vi "MPB_signal_write_read.vi"(8 "error in":errorcluster, 10 "Send Commands":T4, 11 "RBS session in":T1) -> (0 "error out":errorcluster, 2 "MPB Status":T3 {"InletDCportNegLowRes (VDCportNeg)" format="%.2f"; "HeatgActv (HVIL FB)" format="%.2f"; "InletACportEgy (ACfuseNeg)" format="%.2f"; "InletDCportPosLowRes (VDCportPos)" format="%.2f"; "InletACportFuseLowRes (ACfusePos)" format="%.2f"; "DCbusVoltgUpprHalf" format="%.2f"; "Vac" format="%.2f"; "TrfmrTemp2" format="%.2f"; "TrfmrTemp1" format="%.2f"; "HAPSFltCode" format="%.2f"; "ACCurr4" format="%.2f"; "ACCurr3" format="%.2f"; "ACCurr2" format="%.2f"; "ACCurr1" format="%.2f"; "HAPSCurr" format="%.2f"; "HAPSFltFlag" format="%.2f"; "HAPSVoltgOut" format="%.2f"; "HwFltCode" format="%.2f"; "HwFltFlag" format="%.2f"; "HAPSVoltgIn" format="%.2f"; "BattPortPosFuseLowRes" format="%.2f"; "BattPortNegFuseLowRes" format="%.2f"; "BattPortVoltgLowRes" format="%.2f"; "DCbusVoltg" format="%.2f"; "DCbusVoltgLowrHalf" format="%.2f"; "InletDCportVoltgHiRes" format="%.2f"; "BattPortPower" format="%.2f"; "BattVoltgHiRes" format="%.2f"; "BattCurrDAB2" format="%.2f"; "BattCurrDAB1" format="%.2f"}, 3 "RBS session out":T1)   [LabVIEW 2020]
uses:
  controls/Send Commands.ctl
  controls/MPB Status.ctl
  <vilib>/AKKA/PROVEtech-RBS/private/RBS Session.ctl
  <vilib>/AKKA/PROVEtech-RBS/private/RBS Core/RBS Core Data.ctl
  <vilib>/AKKA/PROVEtech-RBS/private/RBS status.ctl
  <vilib>/AKKA/PROVEtech-RBS/SubVIs/Write (Signals Single-point).vi
  <vilib>/AKKA/PROVEtech-RBS/SubVIs/Read (Signals Single-point).vi
  <vilib>/AKKA/PROVEtech-RBS/PROVEtechRBS.lvlib
panel:
  # "Other"
  # "AC Port Info"
  # "Battery Port Info"
  # "Fault Info"
  # "1"
  # "2"
  # "3"
  # "4"
  # "5"
  # "6"
  # "7"
  # "DC Bus Info"
  # "HAPS Info"
  # "Temps"
  # "1"
  # "2"
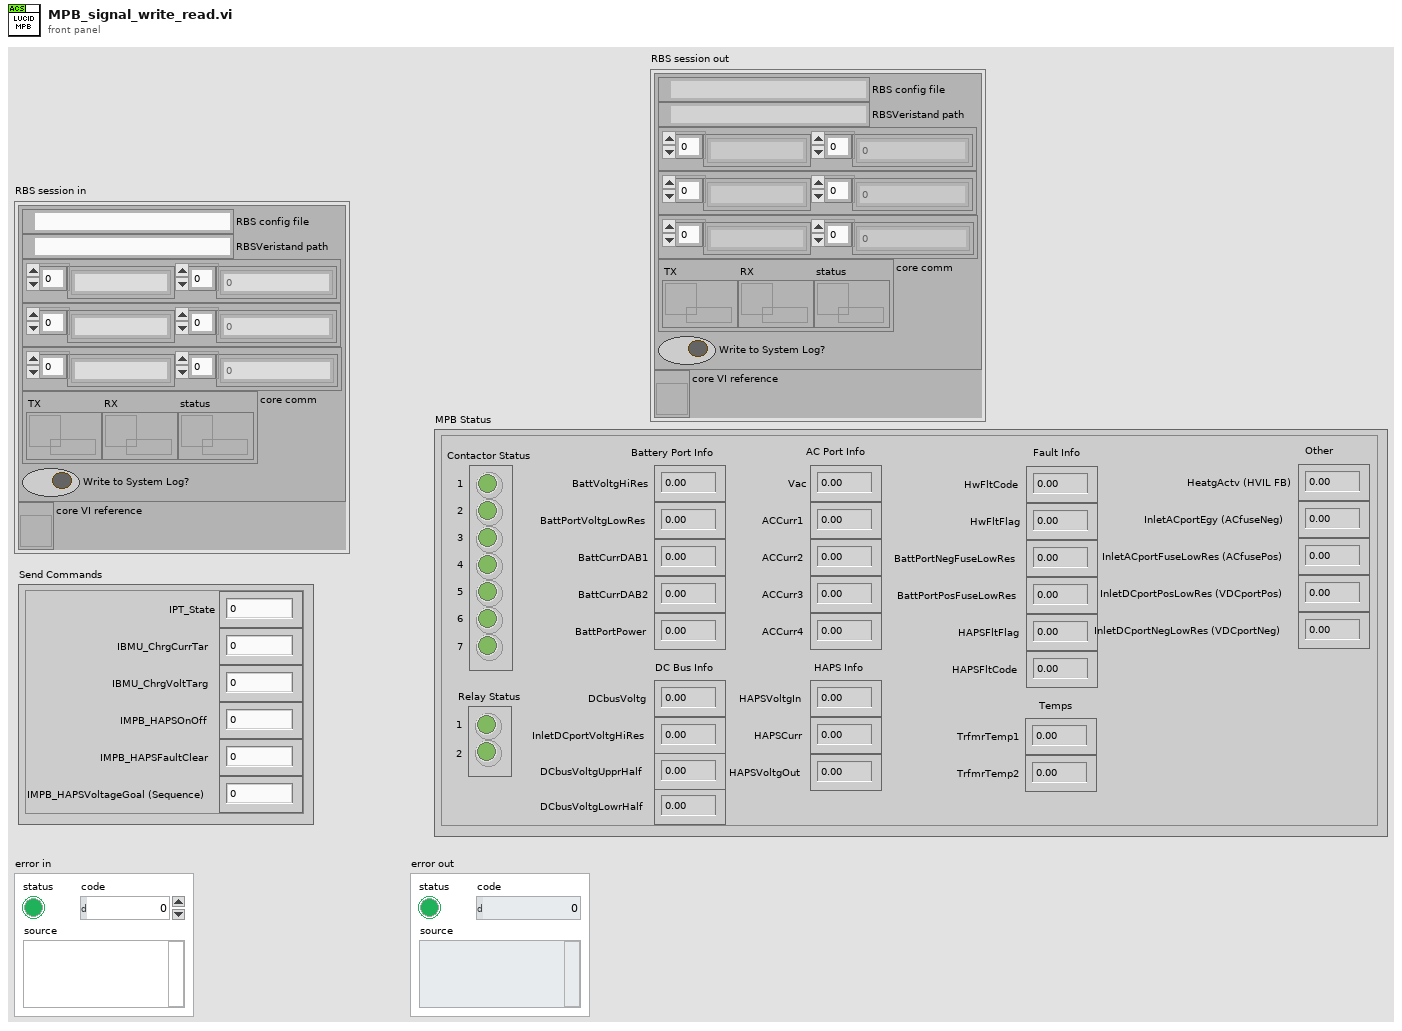
[diagram p1: front panel]
types:
  T1 = typedef "PROVEtechRBS.lvlib/RBS Session.ctl" = cluster{"core":T2, "core VI reference":refnum<vi>}
  T2 = typedef "PROVEtechRBS.lvlib/RBS Core Data.ctl" = cluster{"RBS config file":path, "RBSVeristand path":path, "TX signals":cluster{"names":string[], "values":dbl[]}, "RX signals":cluster{"names":string[], "values":dbl[]}, "TX_enable signals":cluster{"names":string[], "indices":i32[]}, "core comm":cluster{"TX":refnum<data-value>, "RX":refnum<data-value>, "status":refnum<data-value>}, "Write to System Log?":bool}
  T3 = typedef "MPB Status.ctl" = cluster{"Contactor Status":bool[], "Relay Status":bool[], "BattCurrDAB1":dbl, "BattCurrDAB2":dbl, "BattVoltgHiRes":dbl, "BattPortPower":dbl, "InletDCportVoltgHiRes":dbl, "DCbusVoltgLowrHalf":dbl, "DCbusVoltg":dbl, "BattPortVoltgLowRes":dbl, "BattPortNegFuseLowRes":dbl, "BattPortPosFuseLowRes":dbl, "HAPSVoltgIn":dbl, "HwFltFlag":dbl, "HwFltCode":dbl, "HAPSVoltgOut":dbl, "HAPSFltFlag":dbl, "HAPSCurr":dbl, "ACCurr1":dbl, "ACCurr2":dbl, "ACCurr3":dbl, "ACCurr4":dbl, "HAPSFltCode":dbl, "TrfmrTemp1":dbl, "TrfmrTemp2":dbl, "Vac":dbl, "DCbusVoltgUpprHalf":dbl, "InletACportFuseLowRes (ACfusePos)":dbl, "InletDCportPosLowRes (VDCportPos)":dbl, "InletACportEgy (ACfuseNeg)":dbl, "HeatgActv (HVIL FB)":dbl, "InletDCportNegLowRes (VDCportNeg)":dbl}
  T4 = typedef "Send Commands.ctl" = cluster{"IPT_State":dbl, "IBMU_ChrgCurrTar":dbl, "IBMU_ChrgVoltTarg":dbl, "IMPB_HAPSOnOff":dbl, "IMPB_HAPSFaultClear":dbl, "IMPB_HAPSVoltageGoal (Sequence)":dbl}
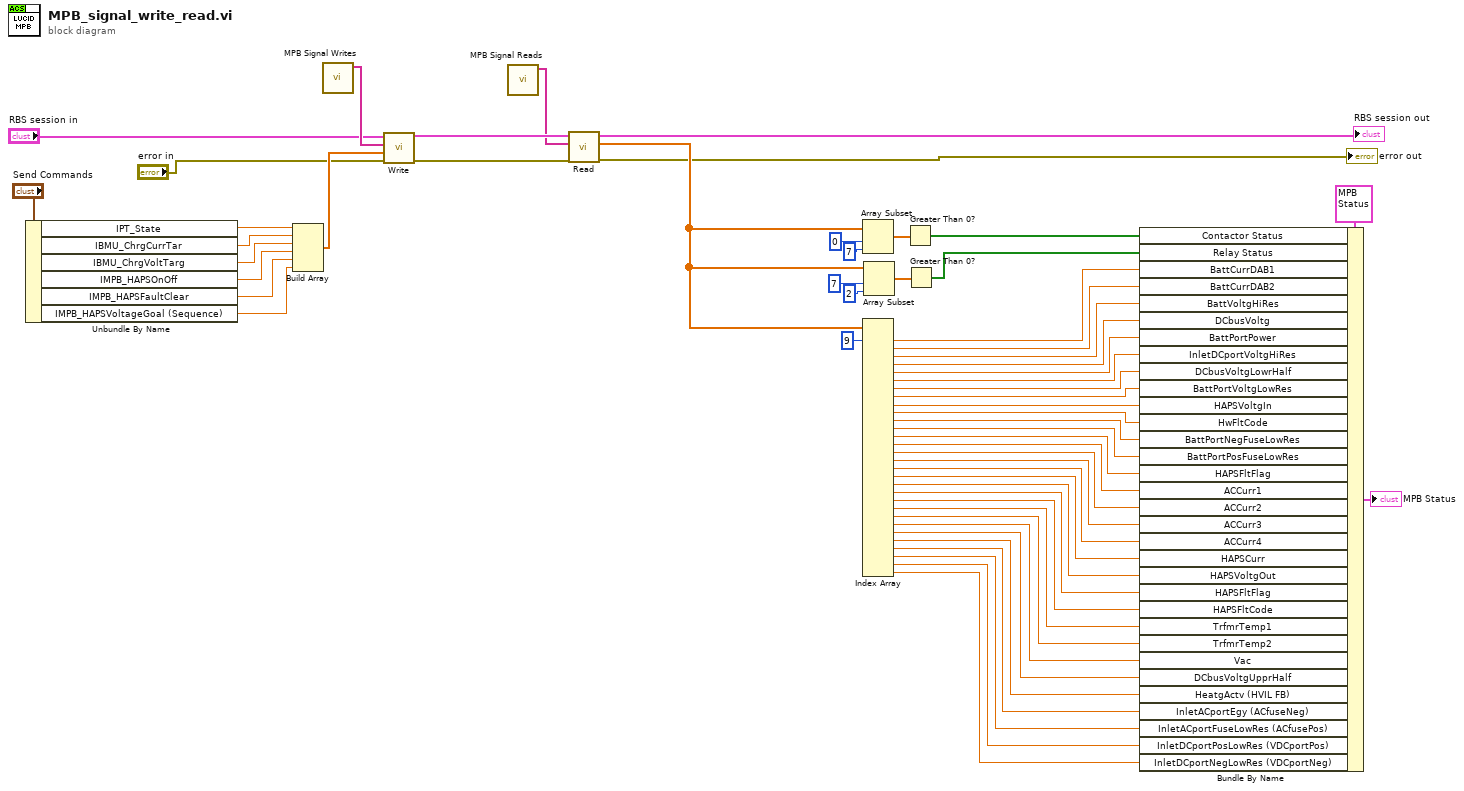
[diagram p0: block diagram]
diagram:
  n1 = Unbundle By Name("Send Commands") -> ("IPT_State"=w57:dbl, "IBMU_ChrgCurrTar"=w17:dbl, "IBMU_ChrgVoltTarg"=w16:dbl, "IMPB_HAPSOnOff"=w18:dbl, "IMPB_HAPSFaultClear"=w19:dbl, "IMPB_HAPSVoltageGoal (Sequence)"=w6:dbl)
  n2 = Build Array(w57, w17, w16, w18, w19, w6) -> (w56:dbl[])
  n3 = call "MPB Signal Writes.vi"() -> ("TX Signals"=w20:string[])  [unwired: 11 in]
  n4 = call-poly <vilib>:"Write.vi"("error in (no error)"="error in", "values"=w56, "signals"=w20, "RBS session in"="RBS session in") -> ("error out"=w55:errorcluster, "RBS session out"=w54:T1)  [unwired: 6 in]
  n5 = call "MPB Signal Reads.vi"() -> ("RX Signals"=w53:string[])  [unwired: 11 in]
  n6 = call-poly <vilib>:"Read.vi"("error in (no error)"=w55, "signals"=w53, "RBS session in"=w54) -> ("error out"=→"error out":errorcluster, "values"=w43:dbl[], "RBS session out"=→"RBS session out":T1)  [unwired: 6 in]
  n7 = Array Subset(array=w43, index=0, length=7) -> (w46:dbl[])
  n8 = Index Array(array=w43, index #1=9 ("index")) -> (element #1=w41:dbl, element #2=w40:dbl, element #3=w39:dbl, element #4=w38:dbl, element #5=w37:dbl, element #6=w36:dbl, element #7=w35:dbl, element #8=w34:dbl, element #9=w33:dbl, element #10=w32:dbl, element #11=w31:dbl, element #12=w30:dbl, element #13=w29:dbl, element #14=w28:dbl, element #15=w27:dbl, element #16=w26:dbl, element #17=w25:dbl, element #18=w24:dbl, element #19=w23:dbl, element #20=w22:dbl, element #21=w21:dbl, element #22=w15:dbl, element #23=w14:dbl, element #24=w13:dbl, element #25=w12:dbl, element #26=w11:dbl, element #27=w10:dbl, element #28=w9:dbl, element #29=w8:dbl, element #30=w7:dbl)  [unwired: 29 in]
  n9 = Array Subset(array=w43, index=7, length=2) -> (w45:dbl[])
  n10 = Greater Than 0?(x=w46) -> (x > 0?=w5:bool[])
  n11 = Greater Than 0?(x=w45) -> (x > 0?=w44:bool[])
  n12 = Bundle By Name(cluster=T3 {"Contactor Status"=[], "Relay Status"=[], "BattCurrDAB1"=0.0, "BattCurrDAB2"=0.0, "BattVoltgHiRes"=0.0, "BattPortPower"=0.0, "InletDCportVoltgHiRes"=0.0, "DCbusVoltgLowrHalf"=0.0, "DCbusVoltg"=0.0, "BattPortVoltgLowRes"=0.0, "BattPortNegFuseLowRes"=0.0, "BattPortPosFuseLowRes"=0.0, "HAPSVoltgIn"=0.0, "HwFltFlag"=0.0, "HwFltCode"=0.0, "HAPSVoltgOut"=0.0, "HAPSFltFlag"=0.0, "HAPSCurr"=0.0, "ACCurr1"=0.0, "ACCurr2"=0.0, "ACCurr3"=0.0, "ACCurr4"=0.0, "HAPSFltCode"=0.0, "TrfmrTemp1"=0.0, "TrfmrTemp2"=0.0, "Vac"=0.0, "DCbusVoltgUpprHalf"=0.0, "InletACportFuseLowRes (ACfusePos)"=0.0, "InletDCportPosLowRes (VDCportPos)"=0.0, "InletACportEgy (ACfuseNeg)"=0.0, "HeatgActv (HVIL FB)"=0.0, "InletDCportNegLowRes (VDCportNeg)"=0.0} ("MPB Status"), "Contactor Status"=w5, "Relay Status"=w44, "BattCurrDAB1"=w41, "BattCurrDAB2"=w40, "BattVoltgHiRes"=w39, "DCbusVoltg"=w38, "BattPortPower"=w37, "InletDCportVoltgHiRes"=w36, "DCbusVoltgLowrHalf"=w35, "BattPortVoltgLowRes"=w34, "HAPSVoltgIn"=w33, "HwFltCode"=w32, "BattPortNegFuseLowRes"=w31, "BattPortPosFuseLowRes"=w30, "HAPSFltFlag"=w29, "ACCurr1"=w28, "ACCurr2"=w27, "ACCurr3"=w26, "ACCurr4"=w25, "HAPSCurr"=w24, "HAPSVoltgOut"=w23, "HAPSFltFlag"=w22, "HAPSFltCode"=w21, "TrfmrTemp1"=w15, "TrfmrTemp2"=w14, "Vac"=w13, "DCbusVoltgUpprHalf"=w12, "HeatgActv (HVIL FB)"=w11, "InletACportEgy (ACfuseNeg)"=w10, "InletACportFuseLowRes (ACfusePos)"=w9, "InletDCportPosLowRes (VDCportPos)"=w8, "InletDCportNegLowRes (VDCportNeg)"=w7) -> (→"MPB Status":T3)
